vi "Noeway_Flashing.vi"(8 "error in (no error)":errorcluster) -> (0 "error in (out)":errorcluster)   [LabVIEW 2024, in "Neoway_flashing.lvlib"]
doc: "This template is for the Queued Message Handler design pattern.\n\nThe Event Handling Loop generates messages based on user interface actions.\n\nThe Message Handling Loop processes messages generated by the Event Handling Loop, or by other messages. The messages are string values, so new messages can be added easily to the Message Cases case structure in the Message Handling Loop. Each message cluster can also provide an optional value for Message Data, which is a variant that can be converted to whatever message-specific data is required."
uses:
  Neoway_flashing.lvlib
  support/Neoway_ctrl.ctl
  controls/Neoway UI Data.ctl
  PrivateControls/FGV_Queue_Control.ctl
  Launcher/SubVI/Global 1.vi
  <vilib>/Utility/error.llb/Error Cluster From Error Code.vi
  <vilib>/ErrorRing/Error Ring.xnode
  support/Message Queue/Neoway Message Queue.lvlib
  support/User Event - Stop/72-13360 User Event - Stop.lvlib
  Launcher/Launcher_DTU.lvlib
panel:
  out "return code":i32
  out "standard output":string
  out "Timer":u32
  in  "Neoway Flashing":T1
  in  "Config":string
  in  "DUT":string
  in  "Read_Res":bool
  in  "Read_Current":bool
  in  "Read_File":bool
  in  "Flash":bool
  out "queue name 2":string
  out "queue name":string
  out "Display <Replace Me>":string
  in  "Output":bool
  in  "Init_Neoway":bool
  in  "Exit":bool
  # "These controls have associated \"Value Changed\" events configured in the Event Structure on the diagram.\n\nReplace them (and reconfigure the Event Structure) with the controls you need for your application."
  # "This template is for the Queued Message Handler design pattern.\n\nSee the block diagram for more information on how to use this template."
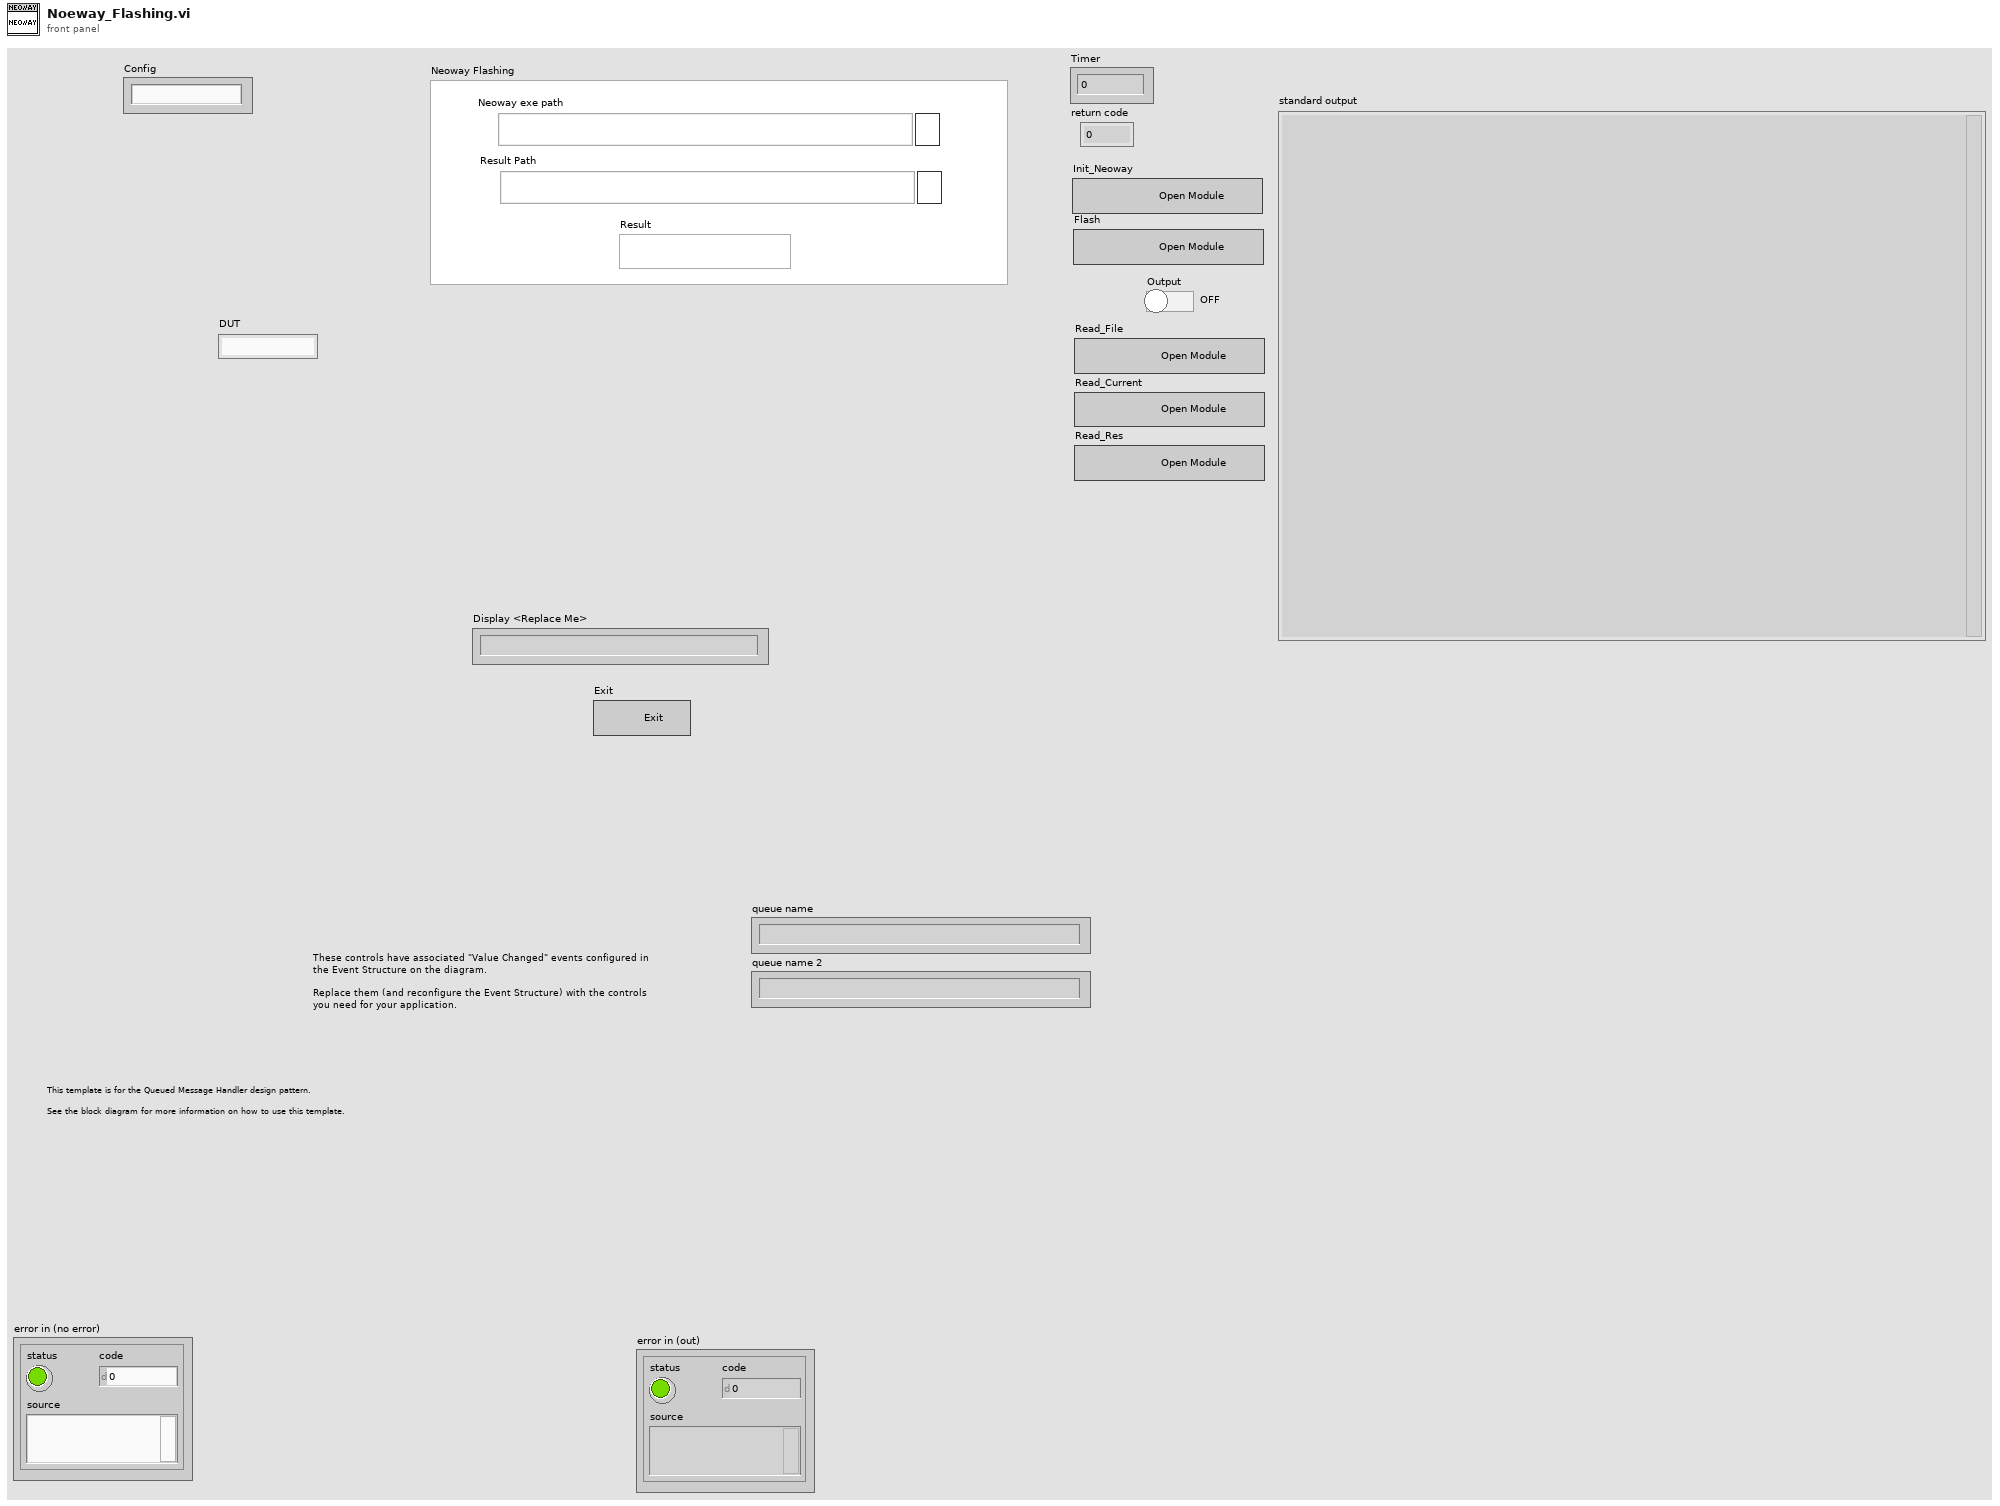
[diagram p1: front panel]
types:
  T1 = typedef "Neoway_flashing.lvlib/Neoway_ctrl.ctl" = cluster{"Neoway exe path":path, "Result Path":path, "Result":string}
  T2 = typedef "Neoway_flashing.lvlib/Neoway UI Data.ctl" = cluster{"DUT":string, "Neoway_Q":refnum<queue>, "notifier out":refnum<notifier>, "Config":string, "Neoway Flashing":T1, "Bat file path":path, "Exe path":string, "Flash path":string, "Timer":u32, "PAC File":string, "CMDDloader":string, "COM":string, "PAC folder":string}
  T3 = typedef "Neoway_flashing.lvlib/FGV_Queue_Control.ctl" = enum16{"Release", "Get", "Set"}
  T4 = typedef "Neoway_flashing.lvlib/Neoway Message Queue.lvlib/All Message Queues.ctl" = cluster{"UI":refnum<queue>, "QSM":refnum<queue>}
  T5 = cluster{"Message":string, "Message Data":variant}
  T6 = enum16{"Read", "Write", "All_sections", "All_values", "Remove key&section"}
  T7 = enum16{"open", "replace", "create", "open or create", "replace or create", "replace or create with confirmation"}
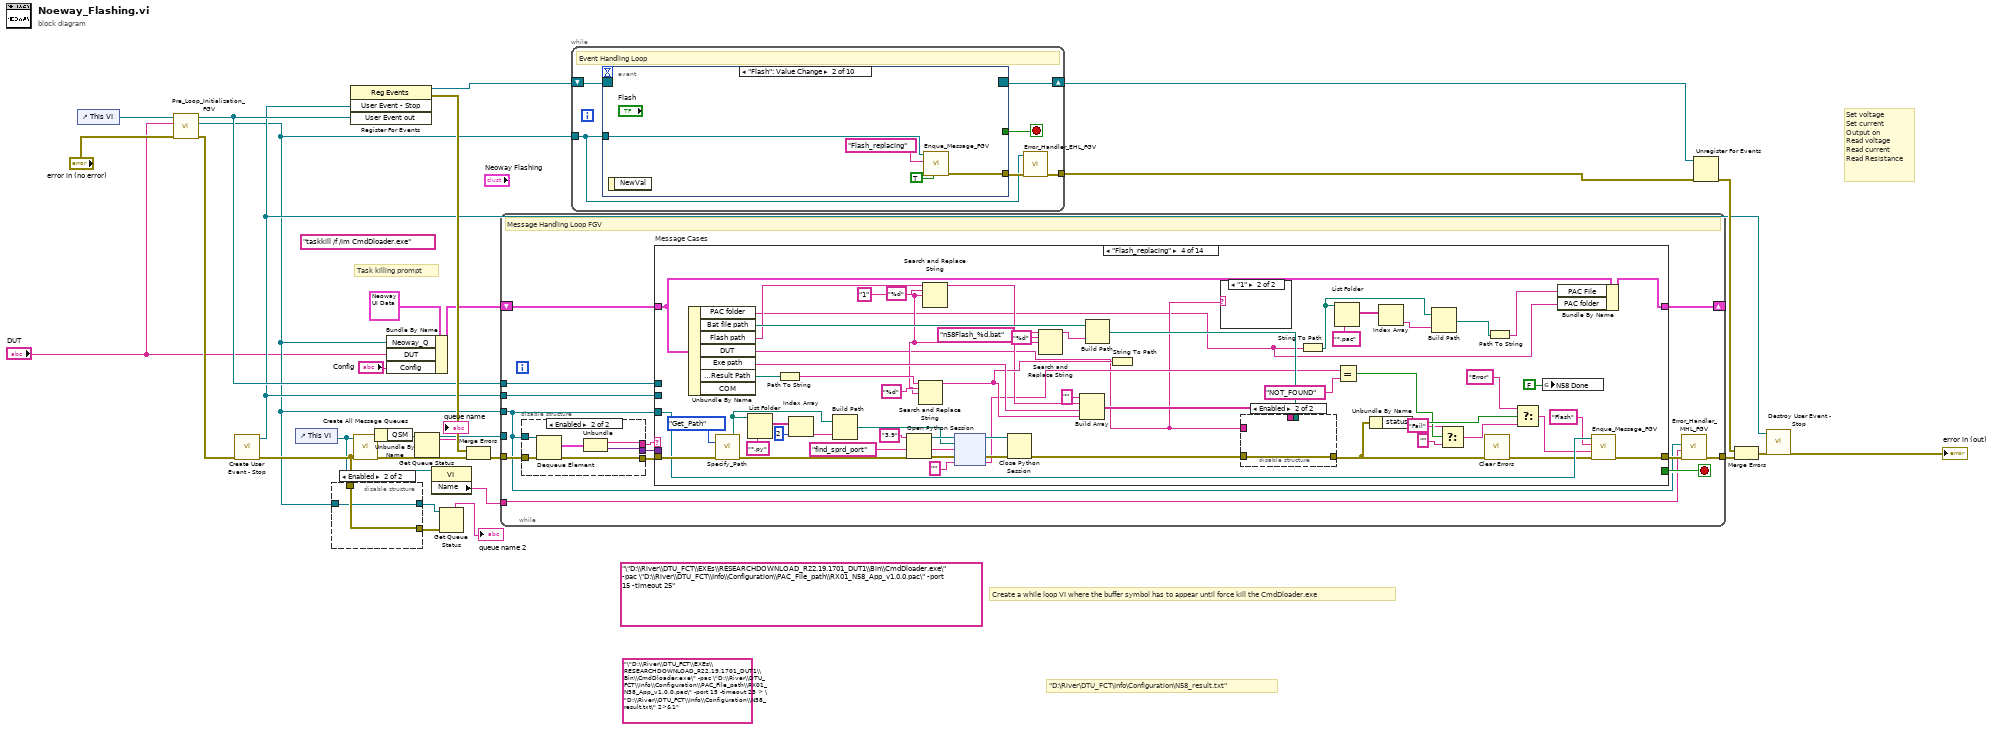
[diagram p0: block diagram]
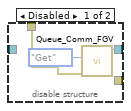
[diagram p2: hidden frame]
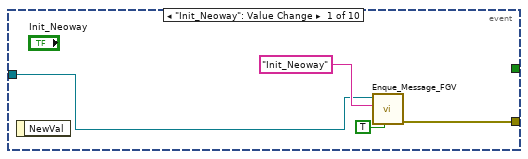
[diagram p3: hidden frame]
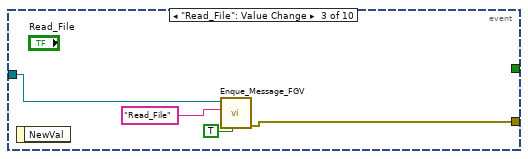
[diagram p4: hidden frame]
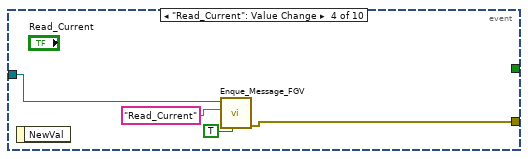
[diagram p5: hidden frame]
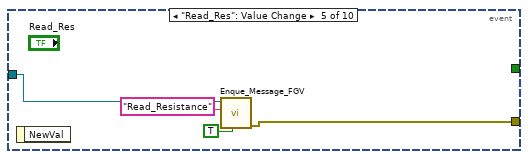
[diagram p6: hidden frame]
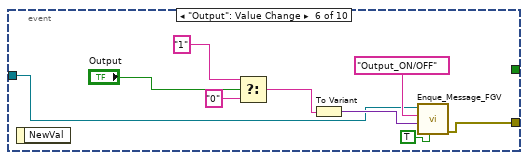
[diagram p7: hidden frame]
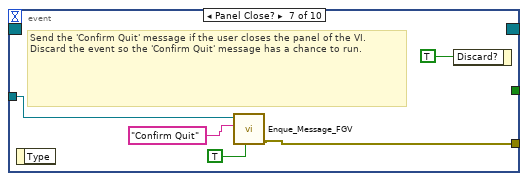
[diagram p8: hidden frame]
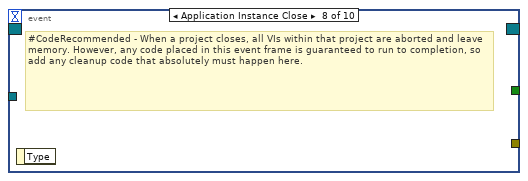
[diagram p9: hidden frame]
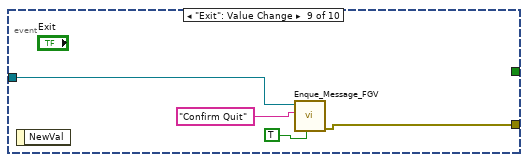
[diagram p10: hidden frame]
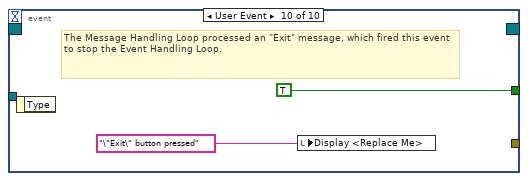
[diagram p11: hidden frame]
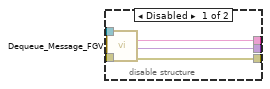
[diagram p12: hidden frame]
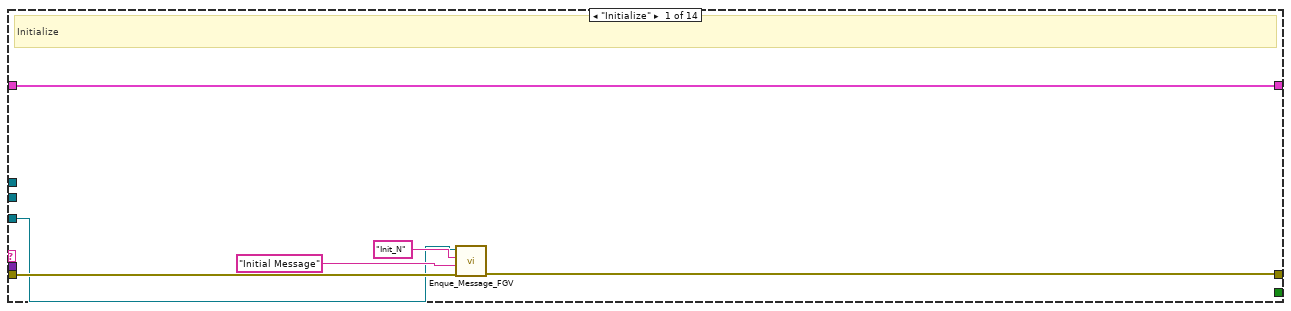
[diagram p13: hidden frame]
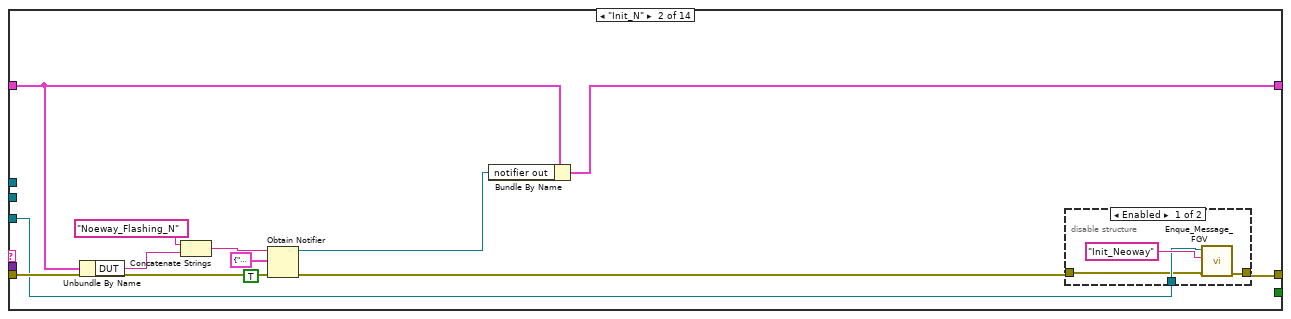
[diagram p14: hidden frame]
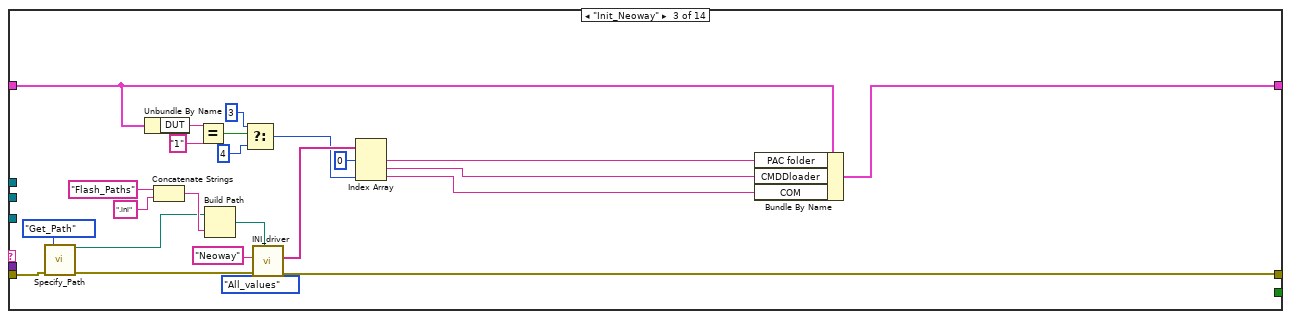
[diagram p16: hidden frame]
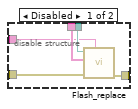
[diagram p18: hidden frame]
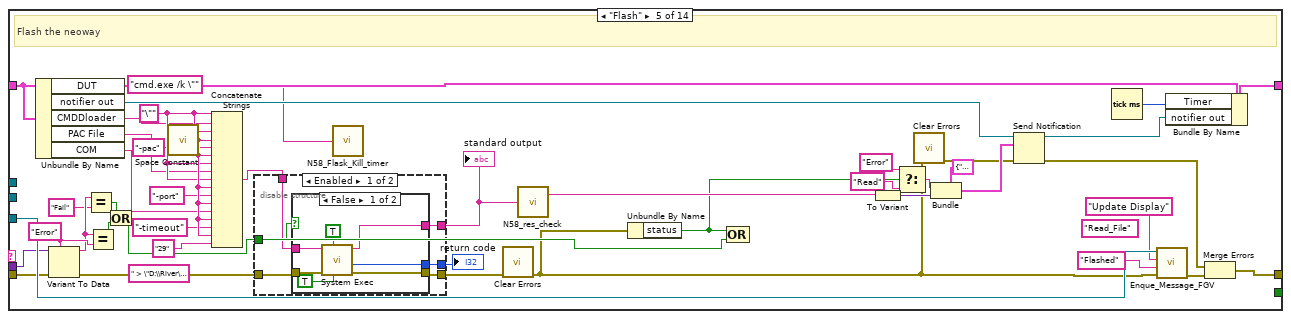
[diagram p19: hidden frame]
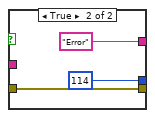
[diagram p20: hidden frame]
diagram:
  (unwired) "\"D:\\River\\DTU_FCT\\EXEs\\RESEARCHDOWNLOAD_R22.19.1701_DUT1\\Bin\\CmdDloader.exe\" -pac \"D:\\River\\DTU_FCT\\Info\\Configuration\\PAC_File_path\\RX01_N58_App_v1.0.0.pac\" -port 15 -timeout 25 > \"D:\\River\\DTU_FCT\\Info\\Configuration\\N58_result.txt\" 2>&1" ("command line")
  (unwired) "\"D:\\River\\DTU_FCT\\EXEs\\RESEARCHDOWNLOAD_R22.19.1701_DUT1\\Bin\\CmdDloader.exe\" -pac \"D:\\River\\DTU_FCT\\Info\\Configuration\\PAC_File_path\\RX01_N58_App_v1.0.0.pac\" -port 15 -timeout 25" ("command line")
  (unwired) "taskkill /f /im CmdDloader.exe"
  # "\"D:\\River\\DTU_FCT\\Info\\Configuration\\N58_result.txt\""
  # "Create a while loop VI where the buffer symbol has to appear until force kill the CmdDloader.exe"
  # "Task killing prompt"
  # "Set voltage\nSet current\nOutput on\nRead voltage \nRead current\nRead Resistance"
  n1 = control-ref of="This VI"() -> (w18:refnum<vi>)
  n2 = call "Pre_Loop_Initialization_FGV.vi"("error in (no error)"="error in (no error)", "DUT"="DUT", "VI in"=w18) -> ("error out"=w16:errorcluster, "queue out"=w5:refnum<queue>, "User Event out"=w9:refnum<user-event>)  [unwired: 6 in]
  n3 = call "Create User Event - Stop.vi"("error in (no error)"=w16) -> ("error out"=w12:errorcluster, "User Event - Stop"=w8:refnum<user-event>)  [unwired: 9 in]
  n4 = control-ref of="This VI"() -> (w2:refnum<vi>)
  n5 = disable-structure shown="Enabled" {
    disable-tunnel: w12 -> [w33 w35]
    disable-tunnel: [w31 w34] -> w11
    disable-tunnel: [_ w35] -> w7
    disable-tunnel: w5 -> [_ w34]
    frame Disabled {
      n6 = call "Queue_Comm_FGV.vi"("error in (no error)"=w33, "Enum"=FGV_Queue_Control."Get") -> ("queue Out"=w31:refnum<queue>)  [unwired: 8 in, 1 out]
    }
    frame Enabled {
    }
  }
  n7 = register-events(w8, w9) -> (reference out=w21:refnum<event-registration>, error out=w19:errorcluster)  [unwired: 2 in]
  n8 = call "Create All Message Queues.vi"("error in (no error)"=w12, "This VI"=w2) -> ("error out"=w30:errorcluster, "Message Queues out"=w29:T4)  [unwired: 8 in]
  n9 = Unbundle By Name(w29) -> ("QSM"=w27:refnum<queue>)
  n10 = Bundle By Name(cluster=T2 {"DUT"="", "Neoway_Q"=refnum, "notifier out"=refnum, "Config"="", "Neoway Flashing"={"Neoway exe path"=path "", "Result Path"=path "", "Result"=""}, "Bat file path"=path "", "Exe path"="", "Flash path"="", "Timer"=0, "PAC File"="", "CMDDloader"="", "COM"="", "PAC folder"=""} ("Data Cluster"), "Neoway_Q"=w5, "DUT"="DUT", "Config"="Config") -> (w6:T2)
  n11 = Get Queue Status(queue=w27) -> (queue out=w14:refnum<queue>, queue name=→"queue name":string)  [unwired: 2 in, 6 out]
  n12 = property class="VI"(reference=w2) -> ("Name"=w1:string)  [unwired: 1 in, 2 out]
  n13 = Get Queue Status(queue=w11, error in (no error)=w7) -> (queue name=→"queue name 2":string)  [unwired: 1 in, 7 out]
  n14 = Merge Errors(w19, w30) -> (w20:errorcluster)
  n15 = while {
    tunnel: w14 -> [_]
    shift-right: [w47] -> _
    shift-left: w6 -> [w48]
    tunnel: w9 -> [w45]
    tunnel: w20 -> [w44]
    tunnel: [w39] -> w28
    tunnel: w8 -> [w38]
    tunnel: w5 -> [w37]
    tunnel: w1 -> [w36]
    stop <- w46 stop-if-true
    # "Message Handling Loop FGV"
    n16 = disable-structure shown="Enabled" {
      disable-tunnel: w44 -> [w52 w58]
      disable-tunnel: [w51 w56] -> w43
      disable-tunnel: [w50 w53] -> w42
      disable-tunnel: [w49 w54] -> w41
      disable-tunnel: w37 -> [_ w57]
      frame Disabled {
        n17 = call "Dequeue_Message_FGV.vi"("error in (no error)"=w52) -> ("error out"=w51:errorcluster, "Message Data"=w50:variant, "Message"=w49:string)  [unwired: 8 in]
      }
      frame Enabled {
        n18 = Dequeue Element(queue=w57, error in (no error)=w58) -> (element=w55:T5, error out=w56:errorcluster)  [unwired: 1 in, 2 out]
        n19 = Unbundle(w55) -> ("Message"=w54:string, "Message Data"=w53:variant)
      }
    }
    n20 = case "Message Cases" shown="\"Flash_replacing\"" w41 {
      selector: w41 -> [_ _ _ _ _ _ _ _ _ _ _ _ _ w417]
      tunnel: w43 -> [w60 w76 w105 w163 w210 w276 w368 w374 w378 w386 w395 w400 w408 _]
      tunnel: [w63 w65 w104 w161 w213 w271 w355 w375 w378 w380 w397 w398 w401 w418] -> w40
      tunnel: w48 -> [w64 w74 w92 w160 w209 w274 w367 w376 w377 w385 w392 w399 w403 w419]
      tunnel: [w64 w69 w94 w108 w204 w273 w367 w376 w377 w385 w392 w399 w403 w419] -> w47
      tunnel: [_ _ _ _ _ _ _ _ _ _ _ _ TRUE _] -> w46
      tunnel: w42 -> [_ _ _ _ w206 w270 _ w373 _ w384 _ _ w410 _]
      tunnel: w45 -> [_ _ _ _ _ _ _ _ _ _ _ _ w411 _]
      tunnel: w38 -> [_ _ _ _ _ _ _ _ _ _ _ _ w406 _]
      tunnel: w37 -> [w59 w67 _ w162 w211 w272 w354 _ _ _ w390 _ w402 _]
      frame "Initialize" {
        # "Initialize"
        n21 = call "Enque_Message_FGV.vi"("error in (no error)"=w60, "Message Data"="Initial Message" ("Initial Message"), "Message"="Init_N", "queue in"=w59) -> ("error out"=w63:errorcluster)  [unwired: 7 in]
      }
      frame "Init_N" {
        n22 = Unbundle By Name(w74) -> ("DUT"=w73:string)
        n23 = Concatenate Strings("Noeway_Flashing_N", w73) -> (w72:string)
        n24 = Obtain Notifier(name (unnamed)=w72, notification data type=T5 {"Message"="", "Message Data"=variant} ("notification"), create if not found? (T)=TRUE, error in (no error)=w76) -> (notifier out=w68:refnum<notifier>, error out=w66:errorcluster)  [unwired: 1 out]
        n25 = Bundle By Name(cluster=w74, "notifier out"=w68) -> (w69:T2)
        n26 = disable-structure shown="Enabled" {
          disable-tunnel: w67 -> [w79 _]
          disable-tunnel: w66 -> [w78 w81]
          disable-tunnel: [w77 w81] -> w65
          frame Enabled {
            n27 = call "Enque_Message_FGV.vi"("error in (no error)"=w78, "Message"="Init_Neoway", "queue in"=w79) -> ("error out"=w77:errorcluster)  [unwired: 8 in]
          }
          frame Disabled {
          }
        }
      }
      frame "Init_Neoway" {
        n28 = call "Specify_Path.vi"("Path_Enum"=enum16{"Find_Path", "Get_Path"}."Get_Path", "error in (no error)"=w105) -> ("Configurations"=w93:path, "error out"=w99:errorcluster)  [unwired: 6 in, 6 out]
        n29 = Unbundle By Name(w92) -> ("DUT"=w91:string)
        n30 = Concatenate Strings("Flash_Paths" ("string"), ".ini" ("string")) -> (w101:string)
        n31 = Equal?(x=w91, y="1") -> (x = y?=w87:bool)
        n32 = Build Path(base path=w93, name or relative path=w101) -> (appended path=w100:path)
        n33 = Select(t=3 ("index"), s=w87, f=4) -> (s? t:f=w84:i32)
        n34 = call "INI_driver.vi"("Enum"=T6."All_values", "instrument file path"=w100, "error in (no error)"=w99, "Section"="Neoway") -> ("error out"=w104:errorcluster, "Values out"=w97:string[])  [unwired: 4 in, 2 out]
        n35 = Index Array(array=w97, index #1=0 ("index"), index #3=w84) -> (element #1=w82:string, element #2=w88:string, element #3=w83:string)  [unwired: 1 in]
        n36 = Bundle By Name(cluster=w92, "PAC folder"=w82, "CMDDloader"=w88, "COM"=w83) -> (w94:T2)
      }
      frame "Flash_replacing" {
        w122 = "1" ("replace string (\"\")")
        n37 = Unbundle By Name(w160) -> ("PAC folder"=w106:string, "Bat file path"=w139:path, "Flash path"=w125:string, "DUT"=w114:string, "Exe path"=w133:string, "Neoway Flashing.Result Path"=w131:path)  [unwired: 1 out]
        n38 = call "Specify_Path.vi"("Path_Enum"=enum16{"Find_Path", "Get_Path"}."Get_Path", "error in (no error)"=w163) -> ("stripped path"=w148:path, "error out"=w146:errorcluster)  [unwired: 6 in, 6 out]
        n39 = List Folder(path=w148, pattern="*.py") -> (filenames=w150:string[])  [unwired: 2 in, 3 out]
        n40 = Path To String(path=w131) -> (string=w129:string)
        n41 = Index Array(array=w150, index=2) -> (element=w149:string)
        n42 = Build Path(base path=w148, name or relative path=w149) -> (appended path=w147:path)
        n43 = Open Python Session(python version="3.9" ("Python version"), 3:w146) -> (session out=w159:refnum<k35>, error out=w158:errorcluster)  [unwired: 1 in]
        n44 = Search and Replace String(input string=w129, search string="%d", replace string=w122) -> (result string=w127:string)  [unwired: 5 in, 3 out]
        n45 = Search and Replace String(input string=w125, search string="%d", replace string=w122) -> (result string=w124:string)  [unwired: 5 in, 3 out]
        n46 = node(w159, w147, "find_sprd_port" ("function name"), w158, "") -> (w157:refnum<k35>, w156:errorcluster, w115:string)  [unwired: 2 out]
        n47 = Close Python Session(session in=w157, error in=w156) -> (11:w145:errorcluster)
        n48 = Search and Replace String(input string="n58Flash_%d.bat", search string="%d", replace string=w122) -> (result string=w132:string)  [unwired: 5 in, 3 out]
        n49 = Build Array("" ("element"), w124, w133, w127) -> (w137:string[])
        n50 = Build Path(base path=w139, name or relative path=w132) -> (appended path=w138:path)
        n51 = String To Path(string=w127) -> ()  [unwired: 1 out]
        n52 = case shown="\"1\"" w114 {
          frame "2", Default {
          }
          frame "1" {
          }
        }
        n53 = disable-structure shown="Enabled" {
          disable-tunnel: w145 -> [w168 w169]
          disable-tunnel: [w167 w169] -> w142
          disable-tunnel: w138 -> [w166 _]
          disable-tunnel: w137 -> [w165 _]
          disable-tunnel: w114 -> [w164 _]
          frame Disabled {
            n54 = call "Flash_replace.vi"("DUT"=w164, "error in"=w168, "Array"=w165, "file path (use dialog)"=w166) -> ("error out"=w167:errorcluster)  [unwired: 7 in]
          }
          frame Enabled {
          }
        }
        n55 = String To Path(string=w106) -> (path=w110:path)
        n56 = List Folder(path=w110, pattern="*.pac") -> (filenames=w112:string[])  [unwired: 2 in, 3 out]
        n57 = Equal?(x=w115, y="NOT_FOUND") -> (x = y?=w118:bool)
        n58 = Unbundle By Name(w142) -> ("status"=w120:bool)
        n59 = Index Array(array=w112) -> (element=w111:string)  [unwired: 1 in]
        n60 = Build Path(base path=w110, name or relative path=w111) -> (appended path=w109:path)
        n61 = Select(t="Fail", s=w118, f="") -> (s? t:f=w117:string)
        n62 = call <vilib>:"Clear Errors.vi"("error in (no error)"=w142) -> ("error out"=w144:errorcluster)  [unwired: 5 in, 1 out]
        n63 = Path To String(path=w109) -> (string=w107:string)
        n64 = Select(t="Error" ("Message"), s=w120, f=w117) -> (s? t:f=w140:string)
        n65 = global write "Global 1.vi" "N58 Done"(FALSE ("N58 Done")) -> ()
        n66 = Bundle By Name(cluster=w160, "PAC File"=w107, "PAC folder"=w106) -> (w108:T2)
        n67 = call "Enque_Message_FGV.vi"("error in (no error)"=w144, "Message Data"=w140, "Message"="Flash", "queue in"=w162) -> ("error out"=w161:errorcluster)  [unwired: 7 in]
      }
      frame "Flash" {
        (unwired) "cmd.exe /k \""
        (unwired) " > \"D:\\River\\DTU_FCT\\Info\\Configuration\\N58_result.txt\" 2>&1\""
        w186 = "\"" ("string")
        (unwired) "Read_File" ("Message")
        w205 = "Error" ("Message")
        # "Flash the neoway"
        n68 = Unbundle By Name(w209) -> ("DUT"=w188:string, "notifier out"=w193:refnum<notifier>, "CMDDloader"=w181:string, "PAC File"=w179:string, "COM"=w180:string)
        n69 = Variant To Data(error in=w210, type=w205, Variant=w206) -> (data=w177:string, error out=w207:errorcluster)
        n70 = Equal?(x=w177, y="Fail") -> (x = y?=w175:bool)
        n71 = Equal?(x=w177, y=w205) -> (x = y?=w174:bool)
        n72 = Or(x=w175, y=w174) -> (x .or. y?=w173:bool)
        n73 = call <vilib>:"Space Constant.vi"() -> ("String"=w187:string)
        n74 = Concatenate Strings(w186, w181, w186, w187, "-pac", w187, w186, w179, w186, w187, "-port" ("string"), w187, w180, w187, "-timeout" ("string"), w187, "29" ("string")) -> (w178:string)
        n75 = disable-structure shown="Enabled" {
          disable-tunnel: w178 -> [w219 _]
          disable-tunnel: [w218 w230] -> w194
          disable-tunnel: w207 -> [w217 w230]
          disable-tunnel: w173 -> [w214 _]
          disable-tunnel: [w216 _] -> w190
          disable-tunnel: [w215 _] -> w202
          frame Enabled {
            n76 = case shown="False" w214 {
              tunnel: w219 -> [w226 _]
              tunnel: [w225 w229] -> w218
              tunnel: w217 -> [w224 w229]
              tunnel: [w222 "Error" ("standard output")] -> w216
              tunnel: [w221 114 ("return code")] -> w215
              frame False {
                n77 = call <vilib>:"System Exec.vi"("run minimized? (F)"=TRUE, "wait until completion? (T)"=TRUE, "error in (no error)"=w224, "command line"=w226) -> ("error out"=w225:errorcluster, "return code"=w221:i32, "standard output"=w222:string)  [unwired: 4 in, 1 out]
              }
              frame True {
              }
            }
          }
          frame Disabled {
          }
        }
        "standard output" <- w190
        "return code" <- w202
        n78 = call "N58_Flask_Kill_timer.vi"("DUTin"=w188) -> ()  [unwired: 1 in]
        n79 = call <vilib>:"Clear Errors.vi"("error in (no error)"=w194) -> ("error out"=w170:errorcluster)  [unwired: 5 in, 1 out]
        n80 = call "N58_res_check.vi"("standard output"=w190) -> ("s? t:f"=w189:string)  [unwired: 1 out]
        n81 = Unbundle By Name(w170) -> ("status"=w172:bool)
        n82 = Compound Arithmetic op=OR(w172, w173) -> ()  [unwired: 1 out]
        n83 = To Variant(anything=w189) -> (Variant=w200:variant)
        n84 = Select(t="Error" ("f"), s=w172, f="Read" ("Message")) -> (s? t:f=w201:string)
        n85 = call <vilib>:"Clear Errors.vi"("error in (no error)"=w170) -> ("error out"=w195:errorcluster)  [unwired: 5 in, 1 out]
        n86 = Bundle(cluster=T5 {"Message"="", "Message Data"=variant} ("notification"), "Message"=w201, "Message Data"=w200) -> (w199:T5)
        n87 = Send Notification(notification=w199, notifier=w193, error in (no error)=w195) -> (notifier out=w192:refnum<notifier>, error out=w191:errorcluster)
        n88 = Tick Count (ms)() -> (millisecond timer value=w203:u32)
        n89 = call "Enque_Message_FGV.vi"("error in (no error)"=w170, "Message Data"="Flashed" ("Message"), "Message"="Update Display", "queue in"=w211) -> ("error out"=w212:errorcluster)  [unwired: 7 in]
        n90 = Bundle By Name(cluster=w209, "Timer"=w203, "notifier out"=w192) -> (w204:T2)
        n91 = Merge Errors(w191, w212) -> (w213:errorcluster)
      }
      frame "Read_File" {
        # "Read Voltage"
        n92 = Variant To Data(error in=w276, type="", Variant=w270) -> (data=w267:string, error out=w266:errorcluster)
        n93 = Unbundle By Name(w274) -> ("Timer"=w244:u32, "notifier out"=w258:refnum<notifier>, "Neoway Flashing.Result Path"=w236:path, "DUT"=w231:string)
        n94 = Equal?(x=w267, y="Error" ("\"Do Something\" button pressed")) -> (x = y?=w250:bool)
        n95 = Tick Count (ms)() -> (millisecond timer value=w247:u32)
        n96 = Subtract(x=w247, y=w244) -> (x-y=w246:u32)
        n97 = Strip Path(path=w236) -> (stripped path=w235:path)  [unwired: 1 out]
        n98 = Divide(x=w246, y=u32 1000) -> (x/y=w243:dbl)
        n99 = Open/Create/Replace File(file path (use dialog)=w236, error in=w266) -> (refnum out=w263:refnum<file>, error out=w265:errorcluster)  [unwired: 4 in, 1 out]
        n100 = To Unsigned Long Integer(number=w243) -> (unsigned 32bit integer=w242:u32)
        "Timer" <- w242
        n101 = Build Path(base path=w235, name or relative path="ResearchDownload.exe") -> (appended path=w233:path)
        n102 = Greater Or Equal?(x=w242, y=u32 20) -> (x >= y?=w240:bool)
        n103 = Read from Text File(file (use dialog)=w263, error in=w265) -> (refnum out=w261:refnum<file>, text=w256:string, error out=w264:errorcluster)  [unwired: 2 in, 1 out]
        n104 = Path To String(path=w233) -> (string=w232:string)
        n105 = Close File(refnum=w261, error in=w264) -> (error out=w252:errorcluster)  [unwired: 1 out]
        n106 = Equal?(x=w256, y="") -> (x = y?=w238:bool)
        n107 = Not(x=w240) -> (.not. x?=w237:bool)
        n108 = Unbundle By Name(w252) -> ("status"=w255:bool)
        n109 = And(x=w237, y=w238) -> (x .and. y?=w239:bool)
        n110 = Compound Arithmetic op=AND(w238, w255) -> (w249:bool)
        n111 = Compound Arithmetic op=OR(w250, w249) -> (w248:bool)
        n112 = case shown="False" w248 {
          tunnel: w252 -> [w288 w345]
          tunnel: [w287 w346] -> w259
          tunnel: w258 -> [w286 w348]
          tunnel: [w285 w347] -> w257
          tunnel: w256 -> [w284 _]
          tunnel: w255 -> [w283 _]
          tunnel: w239 -> [w282 _]
          tunnel: [w281 "Reset_File" ("Message")] -> w254
          tunnel: [w280 "" ("\"Do Something\" button pressed")] -> w253
          tunnel: w252 -> [w279 w353]
          tunnel: [w279 w353] -> w251
          tunnel: w232 -> [w278 _]
          tunnel: w231 -> [w277 _]
          frame False {
            n113 = case shown="False" w282 {
              tunnel: w288 -> [w301 w340]
              tunnel: [w300 w340] -> w287
              tunnel: w286 -> [w299 w339]
              tunnel: [w298 w339] -> w285
              tunnel: w284 -> [w291 _]
              tunnel: w283 -> [w297 _]
              tunnel: [w296 "Read_File" ("Message")] -> w281
              tunnel: [w295 "Read_File" ("\"Do Something\" button pressed")] -> w280
              tunnel: w279 -> [w294 _]
              tunnel: w278 -> [w293 _]
              tunnel: w277 -> [w289 _]
              frame False {
                n114 = Not Equal?(x=w291, y="success") -> (x != y?=w292:bool)
                n115 = case shown="True" w292 {
                  tunnel: w301 -> [w311 w330]
                  tunnel: [w309 w328] -> w300
                  tunnel: w299 -> [w308 w327]
                  tunnel: [w307 w326] -> w298
                  tunnel: w297 -> [w306 w325]
                  tunnel: ["Reset_File" ("Message") "Reset_File" ("Message")] -> w296
                  tunnel: ["" ("\"Do Something\" button pressed") "" ("\"Do Something\" button pressed")] -> w295
                  tunnel: w291 -> [w302 _]
                  tunnel: w294 -> [w303 w321]
                  tunnel: w293 -> [_ w322]
                  tunnel: [w303 w319] -> _
                  tunnel: w289 -> [_ w318]
                  frame False {
                    n116 = To Variant(anything=w302) -> (Variant=w316:variant)
                    n117 = Select(t="Error" ("f"), s=w306, f="Read" ("Message")) -> (s? t:f=w317:string)
                    n118 = call <vilib>:"Clear Errors.vi"("error in (no error)"=w311) -> ("error out"=w310:errorcluster)  [unwired: 5 in, 1 out]
                    n119 = Bundle(cluster=T5 {"Message"="", "Message Data"=variant} ("notification"), "Message"=w317, "Message Data"=w316) -> (w315:T5)
                    n120 = Send Notification(notification=w315, notifier=w308, error in (no error)=w310) -> (notifier out=w307:refnum<notifier>, error out=w309:errorcluster)
                  }
                  frame True {
                    n121 = call "n58_manual_status.vi"("error in (no error)"=w321, "Research exe"=w322, "DUT"=w318) -> ("error out"=w319:errorcluster, "Status"=w320:string)  [unwired: 7 in]
                    n122 = To Variant(anything=w320) -> (Variant=w335:variant)
                    n123 = Select(t="Error" ("f"), s=w325, f="Read" ("Message")) -> (s? t:f=w336:string)
                    n124 = call <vilib>:"Clear Errors.vi"("error in (no error)"=w330) -> ("error out"=w329:errorcluster)  [unwired: 5 in, 1 out]
                    n125 = Bundle(cluster=T5 {"Message"="", "Message Data"=variant} ("notification"), "Message"=w336, "Message Data"=w335) -> (w334:T5)
                    n126 = Send Notification(notification=w334, notifier=w327, error in (no error)=w329) -> (notifier out=w326:refnum<notifier>, error out=w328:errorcluster)
                  }
                }
              }
              frame True {
              }
            }
          }
          frame True {
            n127 = To Variant(anything=errorcluster {"status"=TRUE, "code"=0, "source"="Error at N58 Flashing"} ("error constant")) -> (Variant=w352:variant)
            n128 = call <vilib>:"Clear Errors.vi"("error in (no error)"=w345) -> ("error out"=w349:errorcluster)  [unwired: 5 in, 1 out]
            n129 = Bundle(cluster=T5 {"Message"="", "Message Data"=variant} ("notification"), "Message"="Error" ("f"), "Message Data"=w352) -> (w351:T5)
            n130 = Send Notification(notification=w351, notifier=w348, error in (no error)=w349) -> (notifier out=w347:refnum<notifier>, error out=w346:errorcluster)
          }
        }
        n131 = call <vilib>:"Clear Errors.vi"("error in (no error)"=w251) -> ("error out"=w260:errorcluster)  [unwired: 5 in, 1 out]
        n132 = Bundle By Name(cluster=w274, "Timer"=w244, "notifier out"=w257, "Neoway Flashing.Result Path"=w236) -> (w273:T2)
        n133 = call "Enque_Message_FGV.vi"("error in (no error)"=w260, "Message Data"=w253, "Message"=w254, "queue in"=w272) -> ("error out"=w275:errorcluster)  [unwired: 7 in]
        n134 = Merge Errors(w259, w275) -> (w271:errorcluster)
      }
      frame "Reset_File" {
        n135 = Unbundle By Name(w367) -> ("Neoway Flashing.Result Path"=w365:path)
        n136 = Open/Create/Replace File(file path (use dialog)=w365, error in=w368, operation (0:open)=T7."replace") -> (refnum out=w362:refnum<file>, error out=w366:errorcluster)  [unwired: 3 in, 1 out]
        n137 = Read from Text File(file (use dialog)=w362, error in=w366) -> (refnum out=w359:refnum<file>, text=w360:string, error out=w363:errorcluster)  [unwired: 2 in, 1 out]
        n138 = Equal?(x=w360, y="") -> ()  [unwired: 1 out]
        n139 = Close File(refnum=w359, error in=w363) -> (error out=w356:errorcluster)  [unwired: 1 out]
        n140 = call "Enque_Message_FGV.vi"("error in (no error)"=w356, "Message Data"="Resetted Flash file" ("\"Do Something\" button pressed"), "Message"="Update Display", "queue in"=w354) -> ("error out"=w355:errorcluster)  [unwired: 7 in]
      }
      frame "Update Display" {
        # "#CodeRecommended - If you wish to decouple the Message Handling Loop from your user interface, consider creating User Events (like the \"Stop\" event in this VI) to message the Event Handling Loop whenever the user interface needs updating."
        # "Update Display - Convert the message data to a string to display in the Data Display indicator."
        n141 = Variant To Data(error in=w374, type="", Variant=w373) -> (data=→"Display <Replace Me>":string, error out=w371:errorcluster)
        n142 = Merge Errors(w371) -> (w375:errorcluster)
        n143 = global write "Global 1.vi" "N58 Done"(FALSE ("N58 Done")) -> ()
      }
      frame "Reset" {
      }
      frame "Error" {
        # "Error - Display an error dialog. This message is sent by the \"Error Handler\" VIs at the end of other loops in this application."
        n144 = Variant To Data(error in=w386, type=errorcluster {"status"=FALSE, "code"=0, "source"=""} ("error constant"), Variant=w384) -> (data=w382:errorcluster, error out=w381:errorcluster)
        n145 = call <vilib>:"Simple Error Handler.vi"("error in (no error)"=w382) -> ()  [unwired: 4 in, 5 out]
        n146 = call <vilib>:"Clear Errors.vi"("error in (no error)"=w381) -> ("error out"=w379:errorcluster)  [unwired: 5 in, 1 out]
        n147 = Merge Errors(w379) -> (w380:errorcluster)
      }
      frame "Confirm Quit" {
        # "Confirm Quit - Message that can confirm whether or not the user wants to exit the application."
        n148 = Unbundle By Name(w392) -> ("notifier out"=w388:refnum<notifier>)
        n149 = Release Notifier(notifier=w388, force destroy? (F)=TRUE, error in (no error)=w395) -> (error out=w389:errorcluster)  [unwired: 2 out]
        n150 = call <vilib>:"Clear Errors.vi"("error in (no error)"=w389) -> ("error out"=w391:errorcluster)  [unwired: 5 in, 1 out]
        n151 = call "Enque_Message_FGV.vi"("Priority"=TRUE ("Priority Message? (F)"), "error in (no error)"=w391, "Message"="Exit", "queue in"=w390) -> ("error out"=w396:errorcluster)  [unwired: 7 in]
        n152 = Merge Errors(w396) -> (w397:errorcluster)
      }
      frame "---Copy This Frame---" {
        # "Duplicate this frame when creating new messages.  Change this comment in the duplicated frame to describe this message."
        n153 = Merge Errors(w400) -> (w398:errorcluster)
      }
      frame "Exit" {
        # "Stop the VI"
        # "Release the message queue reference"
        # "Exit - Exit the application."
        n154 = disable-structure shown="Disabled" {
          disable-tunnel: w410 -> [w414 _]
          frame Disabled {
            n155 = Variant To Data(type=errorcluster {"status"=FALSE, "code"=0, "source"=""} ("error constant"), Variant=w414) -> (data=w415:errorcluster)  [unwired: 1 in, 1 out]
            n156 = call <vilib>:"Simple Error Handler.vi"("error in (no error)"=w415) -> ()  [unwired: 4 in, 5 out]
          }
          frame Enabled {
          }
        }
        n157 = call "Queue_Comm_FGV.vi"("error in (no error)"=w408, "Enum"=FGV_Queue_Control."Release", "queue in"=w402) -> ("error Out"=w407:errorcluster)  [unwired: 7 in, 1 out]
        n158 = call "Fire User Event - Stop.vi"("User Event - Stop"=w406) -> ("error out"=w404:errorcluster)  [unwired: 10 in]
        n159 = call "Fire User Event - Stop.vi"("User Event - Stop"=w411) -> ("error out"=w405:errorcluster)  [unwired: 10 in]
        n160 = Merge Errors(w405, w404, w407) -> (w412:errorcluster)
        n161 = call <vilib>:"Clear Errors.vi"("error in (no error)"=w412) -> ("error out"=w401:errorcluster)  [unwired: 5 in, 1 out]
      }
      frame Default {
        # "'Default' case only runs if there is a message that isn't defined in any of the other cases.  Output a programming error."
        n162 = xnode "Error Ring"("parameter 0"=w417) -> ("error out"=w418:errorcluster)
      }
    }
    n163 = call "Error_Handler_MHL_FGV.vi"("error in (no error)"=w40, "VI_name"=w36, "queue in"=w37) -> ("error Out"=w39:errorcluster)  [unwired: 8 in]
  }
  n164 = while {
    shift-right: [w431] -> w24
    shift-left: w21 -> [w432]
    tunnel: [w428] -> w22
    tunnel: w5 -> [w427]
    stop <- w430 stop-if-true
    # "Event Handling Loop"
    n165 = event shown="[1] \"Flash\": Value Change" {
      selector: w432 -> [_ _ _ _ _ _ _ _ _ _]
      dyn-events: [_ _ _ _ _ _ _ _ _ _] -> w431
      timeout: _ -> [_ _ _ _ _ _ _ _ _ _]
      tunnel: [_ _ _ _ _ _ _ _ _ TRUE ("Discard?")] -> w430
      tunnel: [w435 w439 w443 w447 w451 w459 w465 _ w470 _] -> w429
      tunnel: w427 -> [w433 w437 w441 w445 w449 w453 w462 _ w467 _]
      event "Init_Neoway": Value Change {
        n166 = event-data() -> ()  [unwired: 1 in, 1 out]
        n167 = call "Enque_Message_FGV.vi"("Priority"=TRUE ("Priority Message? (F)"), "Message"="Init_Neoway", "queue in"=w433) -> ("error out"=w435:errorcluster)  [unwired: 8 in]
      }
      event "Flash": Value Change {
        n168 = event-data() -> ()  [unwired: 1 in, 1 out]
        n169 = call "Enque_Message_FGV.vi"("Priority"=TRUE ("Priority Message? (F)"), "Message"="Flash_replacing", "queue in"=w437) -> ("error out"=w439:errorcluster)  [unwired: 8 in]
      }
      event "Read_File": Value Change {
        n170 = event-data() -> ()  [unwired: 1 in, 1 out]
        n171 = call "Enque_Message_FGV.vi"("Priority"=TRUE ("Priority Message? (F)"), "Message"="Read_File", "queue in"=w441) -> ("error out"=w443:errorcluster)  [unwired: 8 in]
      }
      event "Read_Current": Value Change {
        n172 = event-data() -> ()  [unwired: 1 in, 1 out]
        n173 = call "Enque_Message_FGV.vi"("Priority"=TRUE ("Priority Message? (F)"), "Message"="Read_Current", "queue in"=w445) -> ("error out"=w447:errorcluster)  [unwired: 8 in]
      }
      event "Read_Res": Value Change {
        n174 = event-data() -> ()  [unwired: 1 in, 1 out]
        n175 = call "Enque_Message_FGV.vi"("Priority"=TRUE ("Priority Message? (F)"), "Message"="Read_Resistance", "queue in"=w449) -> ("error out"=w451:errorcluster)  [unwired: 8 in]
      }
      event "Output": Value Change {
        n176 = event-data() -> ()  [unwired: 1 in, 1 out]
        n177 = Select(t="1", s="Output", f="0") -> (s? t:f=w455:string)
        n178 = To Variant(anything=w455) -> (Variant=w454:variant)
        n179 = call "Enque_Message_FGV.vi"("Priority"=TRUE ("Priority Message? (F)"), "Message Data"=w454, "Message"="Output_ON/OFF", "queue in"=w453) -> ("error out"=w459:errorcluster)  [unwired: 7 in]
      }
      event Panel Close? {
        # "Send the 'Confirm Quit' message if the user closes the panel of the VI. Discard the event so the 'Confirm Quit' message has a chance to run."
        n180 = event-data() -> ()  [unwired: 1 in, 1 out]
        n181 = call "Enque_Message_FGV.vi"("Priority"=TRUE ("Priority Message? (F)"), "Message"="Confirm Quit", "queue in"=w462) -> ("error out"=w465:errorcluster)  [unwired: 8 in]
        n182 = event-data("Discard?"=TRUE) -> ()  [unwired: 1 in, 1 out]
      }
      event Application Instance Close {
        # "#CodeRecommended - When a project closes, all VIs within that project are aborted and leave memory. However, any code placed in this event frame is guaranteed to run to completion, so add any cleanup code that absolutely must happen here."
        n183 = event-data() -> ()  [unwired: 1 in, 1 out]
      }
      event "Exit": Value Change {
        n184 = event-data() -> ()  [unwired: 1 in, 1 out]
        n185 = call "Enque_Message_FGV.vi"("Priority"=TRUE ("Priority Message? (F)"), "Message"="Confirm Quit", "queue in"=w467) -> ("error out"=w470:errorcluster)  [unwired: 8 in]
      }
      event User Event {
        # "The Message Handling Loop processed an \"Exit\" message, which fired this event to stop the Event Handling Loop."
        n186 = event-data() -> ()  [unwired: 1 in, 1 out]
        n187 = local write "Display <Replace Me>"("\"Exit\" button pressed" ("VI Stopped")) -> ()
      }
    }
    n188 = call "Error_Handler_EHL_FGV.vi"("error in (no error)"=w429, "queue in"=w427) -> ("error Out"=w428:errorcluster)  [unwired: 9 in]
  }
  n189 = Unregister For Events(event registration refnum=w24, error in=w22) -> (error out=w25:errorcluster)
  n190 = Merge Errors(w25, w28) -> (w26:errorcluster)
  n191 = call "Destroy User Event - Stop.vi"("error in (no error)"=w26, "User Event - Stop"=w8) -> ("error out"=→"error in (out)":errorcluster)  [unwired: 9 in]
